vi "PRIME Move Raw File.vi"(8 "error in":errorcluster, 9 "Source File":path, 10 "Filename":string, 11 "target path":path) -> (0 "error out":errorcluster, 2 "files":path, 3 "This Acq Image Folder":path)   [LabVIEW 2021]
panel:
  out "Moved?":bool
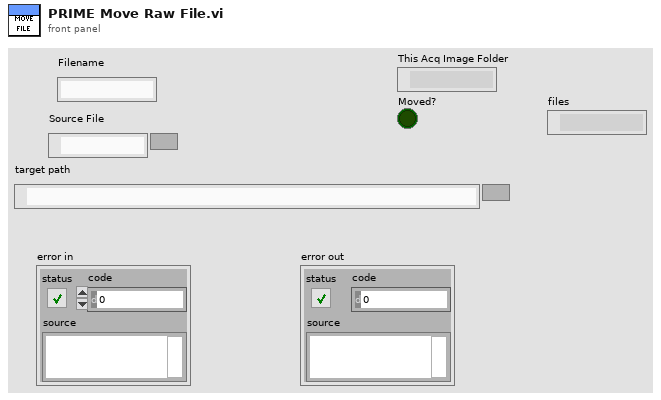
[diagram p1: front panel]
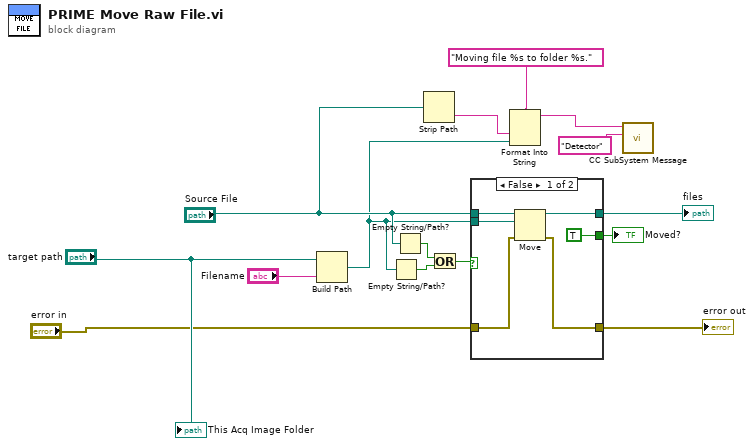
[diagram p0: block diagram]
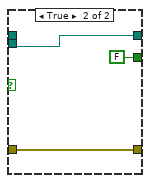
[diagram p2: hidden frame]
diagram:
  n1 = Build Path(base path="target path", name or relative path="Filename") -> (appended path=w5:path)
  n2 = Empty String/Path?(string/path=w5) -> (empty?=w3:bool)
  n3 = Empty String/Path?(string/path="Source File") -> (empty?=w2:bool)
  n4 = Strip Path(path="Source File") -> (name=w8:string)  [unwired: 1 out]
  n5 = Or(x=w2, y=w3) -> (x .or. y?=w4:bool)
  n6 = case shown="False" w4 {
    tunnel: "error in" -> [w21 w23]
    tunnel: [w20 w23] -> w13
    tunnel: [w19 w24] -> w10
    tunnel: w5 -> [w18 w24]
    tunnel: "Source File" -> [w17 _]
    tunnel: [TRUE FALSE] -> w1
    frame False {
      n7 = Move(source path=w17, error in=w21, 10:w18) -> (error out=w20:errorcluster, 3:w19:path)  [unwired: 2 in, 1 out]
    }
    frame True {
    }
  }
  "error out" <- w13
  "files" <- w10
  "Moved?" <- w1
  n8 = Format Into String(format string="Moving file %s to folder %s.", w8, w5) -> (resulting string=w6:string)  [unwired: 2 in, 1 out]
  n9 = call "CC SubSystem Message.vi"("Subsystem"="Detector", "Message"=w6) -> ()  [unwired: 9 in, 1 out]
  "This Acq Image Folder" <- "target path"
